vi "Write FK Column.vi"(8 "error in (no error)":errorcluster, 10 "PK Column":string, 11 "FK Ring in":refnum<class "FK Ring.lvclass">) -> (0 "error out":errorcluster, 3 "FK Ring out":refnum<class "FK Ring.lvclass">)   [LabVIEW 2020, in "FK Ring.lvclass"]
uses:
  FK Ring.lvclass
  FK Ring.lvclass/FK Ring.ctl
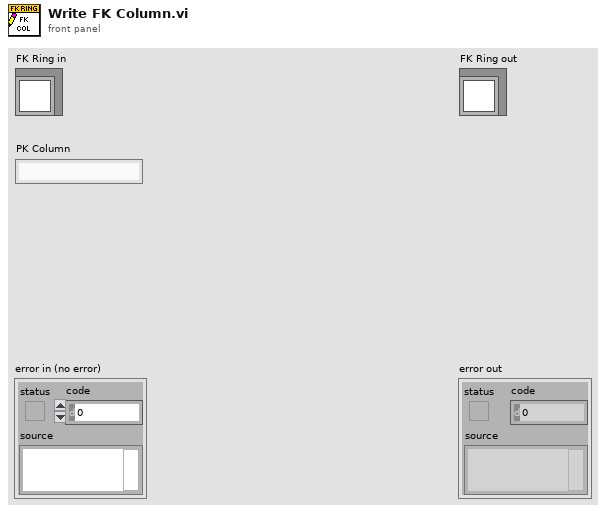
[diagram p1: front panel]
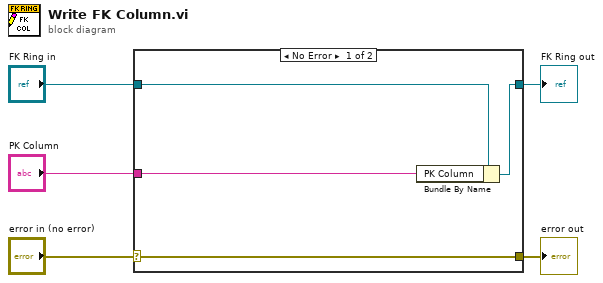
[diagram p0: block diagram]
diagram:
  n1 = case shown="No Error" "error in (no error)" {
    selector: "error in (no error)" -> [w9 w10]
    tunnel: [w9 w10] -> w4
    tunnel: [w7 w11] -> w2
    tunnel: "FK Ring in" -> [w8 w11]
    tunnel: "PK Column" -> [w6 _]
    frame No Error {
      n2 = Bundle By Name(cluster=w8, "PK Column"=w6) -> (w7:refnum<class "FK Ring.lvclass">)
    }
    frame Error {
    }
  }
  "error out" <- w4
  "FK Ring out" <- w2
